vi "Rachel_Wheel_TestV2.vi"(10 "Spin or not to spin":bool, 11 "Oculus Data":T1={"head"={"orientation"={"roll"=1.6327005330047937, "pitch"=-89.08559793078238, "yaw"=-40.95061142092874}, "position"={"x"=1.207441, "y"=0.483058, "z"=-0.742013}}, "hands"={"left"={"position"={"x"=inf, "y"=inf, "z"=-inf}, "orientation"={"roll"=-51.475846117481964, "pitch"=106.93248840397386, "yaw"=69.74254276716579}}, "right"={"position"={"x"=inf, "y"=inf, "z"=-inf}, "orientation"={"roll"=49.02272731762935, "pitch"=105.46319543414037, "yaw"=-123.9602784132463}}}, "buttons"={"a"=FALSE, "b"=FALSE, "x"=FALSE, "y"=FALSE, "menu"=FALSE, "leftTrig"=1e-06, "rightTrig"=1e-06, "leftGrip"=1e-06, "rightGrip"=1e-06, "left_jstick"={"x"=-0.002561, "y"=0.007201, "button"=FALSE}, "right_jstick"={"x"=0.0, "y"=0.0, "button"=FALSE}}}) -> (3 "2D Picture":picture)   [LabVIEW 2017]
uses:
  <vilib>/myRIO/Instrument Drivers/Onboard IO/PWM/typedefs/PWM Reference.ctl
  <vilib>/myRIO/Common/Instrument Driver Framework/Utilities/typedefs/myRIO Generic Hardware Reference.ctl
  <vilib>/myRIO/Common/Instrument Driver Framework/Utilities/typedefs/Hardware Version Enum.ctl
  <vilib>/myRIO/Common/Instrument Driver Framework/Utilities/typedefs/myRIO v1.0 Reference.ctl
  <vilib>/myRIO/Common/Instrument Driver Framework/Utilities/typedefs/Generic FPGA Reference.ctl
  <vilib>/myRIO/Common/Instrument Driver Framework/myRIO v1.0/PWM/typedefs/PWM Channels Enum.ctl
  <vilib>/myRIO/Instrument Drivers/Onboard IO/PWM/typedefs/PWM Configuration.ctl
  <vilib>/userdefined/High Color/nirio_resource_hc.ctl
  <vilib>/myRIO/Common/Instrument Driver Framework/Utilities/vis/Is FPGA Ref Available.vi
  <vilib>/myRIO/Common/Instrument Driver Framework/myRIO v1.0/PWM/vis/myRIO v1.1 Open PWM.vi
  <vilib>/myRIO/Instrument Drivers/Onboard IO/PWM/vis/Set Duty Cycle and Frequency.vi
  <vilib>/myRIO/Common/Instrument Driver Framework/Utilities/vis/Validate Channels.vi
  <vilib>/myRIO/Common/Instrument Driver Framework/myRIO v1.0/PWM/vis/myRIO v1.0 Reserve PWM.vi
  <vilib>/myRIO/Common/Instrument Driver Framework/myRIO v1.0/PWM/vis/myRIO v1.0 Build MUX Configuration PWM.vi
  <vilib>/myRIO/Common/Instrument Driver Framework/myRIO v1.0/Resource Manager/vis/myRIO v1.0 Reserve Channel List.vi
  <vilib>/myRIO/Common/Instrument Driver Framework/myRIO v1.0/Resource Manager/vis/myRIO v1.0 Create Configuration List.vi
  <vilib>/myRIO/Common/Instrument Driver Framework/myRIO v1.0/Resource Manager/vis/myRIO v1.0 Reserve Channel.vi
  <vilib>/myRIO/Common/Instrument Driver Framework/myRIO v1.0/Resource Manager/vis/myRIO v1.0 Unreserve Channel.vi
  <vilib>/myRIO/Common/Instrument Driver Framework/myRIO v1.0/Resource Manager/vis/myRIO v1.0 Build Mutex Name.vi
  <vilib>/Utility/VariantDataType/GetNumericInfo.vi
  <vilib>/Utility/error.llb/Error Cluster From Error Code.vi
  <vilib>/myRIO/Common/Instrument Driver Framework/myRIO v1.0/myRIO v1.1 Open.vi
  <vilib>/myRIO/Common/Instrument Driver Framework/Utilities/vis/IO Manager.vi
  <vilib>/myRIO/Common/Instrument Driver Framework/Utilities/vis/Configuration Manager.vi
  <vilib>/myRIO/Common/Instrument Driver Framework/myRIO v1.0/Resource Manager/vis/myRIO v1.0 Configure IO.vi
  <vilib>/myRIO/Common/Instrument Driver Framework/myRIO v1.0/myRIO v1.0 Close.vi
  <vilib>/myRIO/Common/Instrument Driver Framework/myRIO v1.0/PWM/vis/myRIO v1.0 Write PWM.vi
  <vilib>/express/express arith-compare/Formula/XNode/ExpressFormulaBlockNode.xnode
  <vilib>/myRIO/Express VI/Onboard IO/PWM/PWM Express VI.xnode
  <vilib>/myRIO/Instrument Drivers/Onboard IO/PWM/vis/myRIO PWM Open.xnode
  <vilib>/myRIO/Instrument Drivers/Onboard IO/PWM/PWM.lvlib
panel:
  out "output cluster 2":cluster{dbl, dbl}={149.4878, 198.5598}
  in  "Arrow Size":dbl=15.0 format="%#_13g"
  in  "Rotation Radius":dbl=50.0 format="%#_13g"
  out "max value":dbl=0.007516748932651743
  out "SuMM":dbl(slide)=2.168404344971009e-18 scale=-3.0..3.0
  out "M3 Slider":dbl(slide)=-0.004955748932651739 scale=-1.0..1.0
  out "M2 Slider":dbl(slide)=0.007516748932651743 scale=-1.0..1.0
  out "M1 Slider":dbl(slide)=-0.002561000000000002 scale=-1.0..1.0
  out "r scaled":dbl=0.007642847767684503
  out "Duty 3":dbl=0.075
  out "Duty 2":dbl=0.075
  out "Duty 1":dbl=0.075
  out "buttons.rightGrip":dbl=1e-06
  out "buttons.leftGrip":dbl=1e-06
  out "RightJoyStick X":dbl(slide) scale=-1.0..1.0
  out "X":dbl=-0.002561
  out "theta temp":dbl=1.91249126492638
  out "r":dbl=0.007642847767684503
  out "M 3":dbl=-0.004955748932651739
  out "M 2":dbl=0.007516748932651743
  out "M 1":dbl=-0.002561000000000002
  out "Theta3":dbl=220.4223221640822
  out "Theta2":dbl=100.4223221640822
  out "Theta1":dbl=-19.577677835917797
  out "output cluster":cluster{dbl, dbl}={199.4878, 198.5598}
  out "Phi":dbl=109.5776778359178
  out "alpha3":dbl=330.0
  out "alpha2":dbl=210.0
  out "alpha1":dbl=90.0
  out "Y":dbl=0.007201
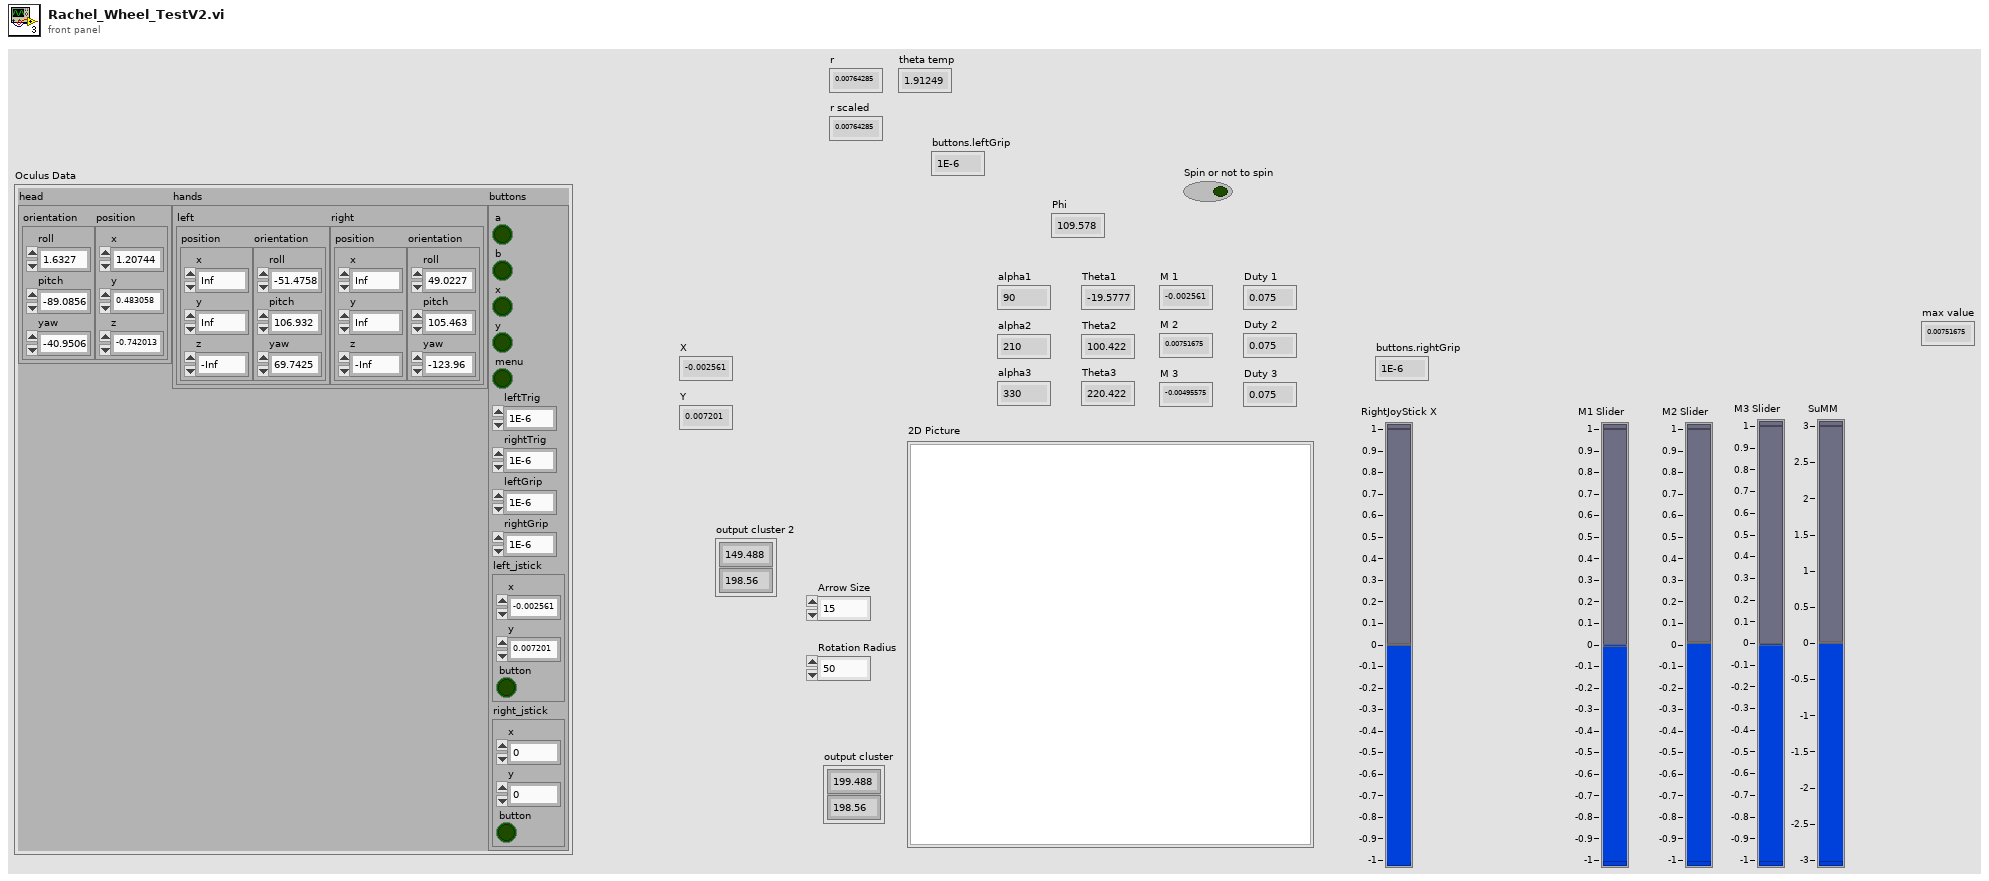
[diagram p1: front panel]
types:
  T1 = cluster{"head":cluster{"orientation":cluster{"roll":dbl, "pitch":dbl, "yaw":dbl}, "position":cluster{"x":dbl, "y":dbl, "z":dbl}}, "hands":cluster{"left":cluster{"position":cluster{"x":dbl, "y":dbl, "z":dbl}, "orientation":cluster{"roll":dbl, "pitch":dbl, "yaw":dbl}}, "right":cluster{"position":cluster{"x":dbl, "y":dbl, "z":dbl}, "orientation":cluster{"roll":dbl, "pitch":dbl, "yaw":dbl}}}, "buttons":cluster{"a":bool, "b":bool, "x":bool, "y":bool, "menu":bool, "leftTrig":dbl, "rightTrig":dbl, "leftGrip":dbl, "rightGrip":dbl, "left_jstick":cluster{"x":dbl, "y":dbl, "button":bool}, "right_jstick":cluster{"x":dbl, "y":dbl, "button":bool}}}
  T2 = cluster{"left":i16, "top":i16, "right":i16, "bottom":i16}
  T3 = cluster{"Width":u16, "Style":enum32{"Solid", "Dash", "Dot", "DashDot", "DashDotDot"}}
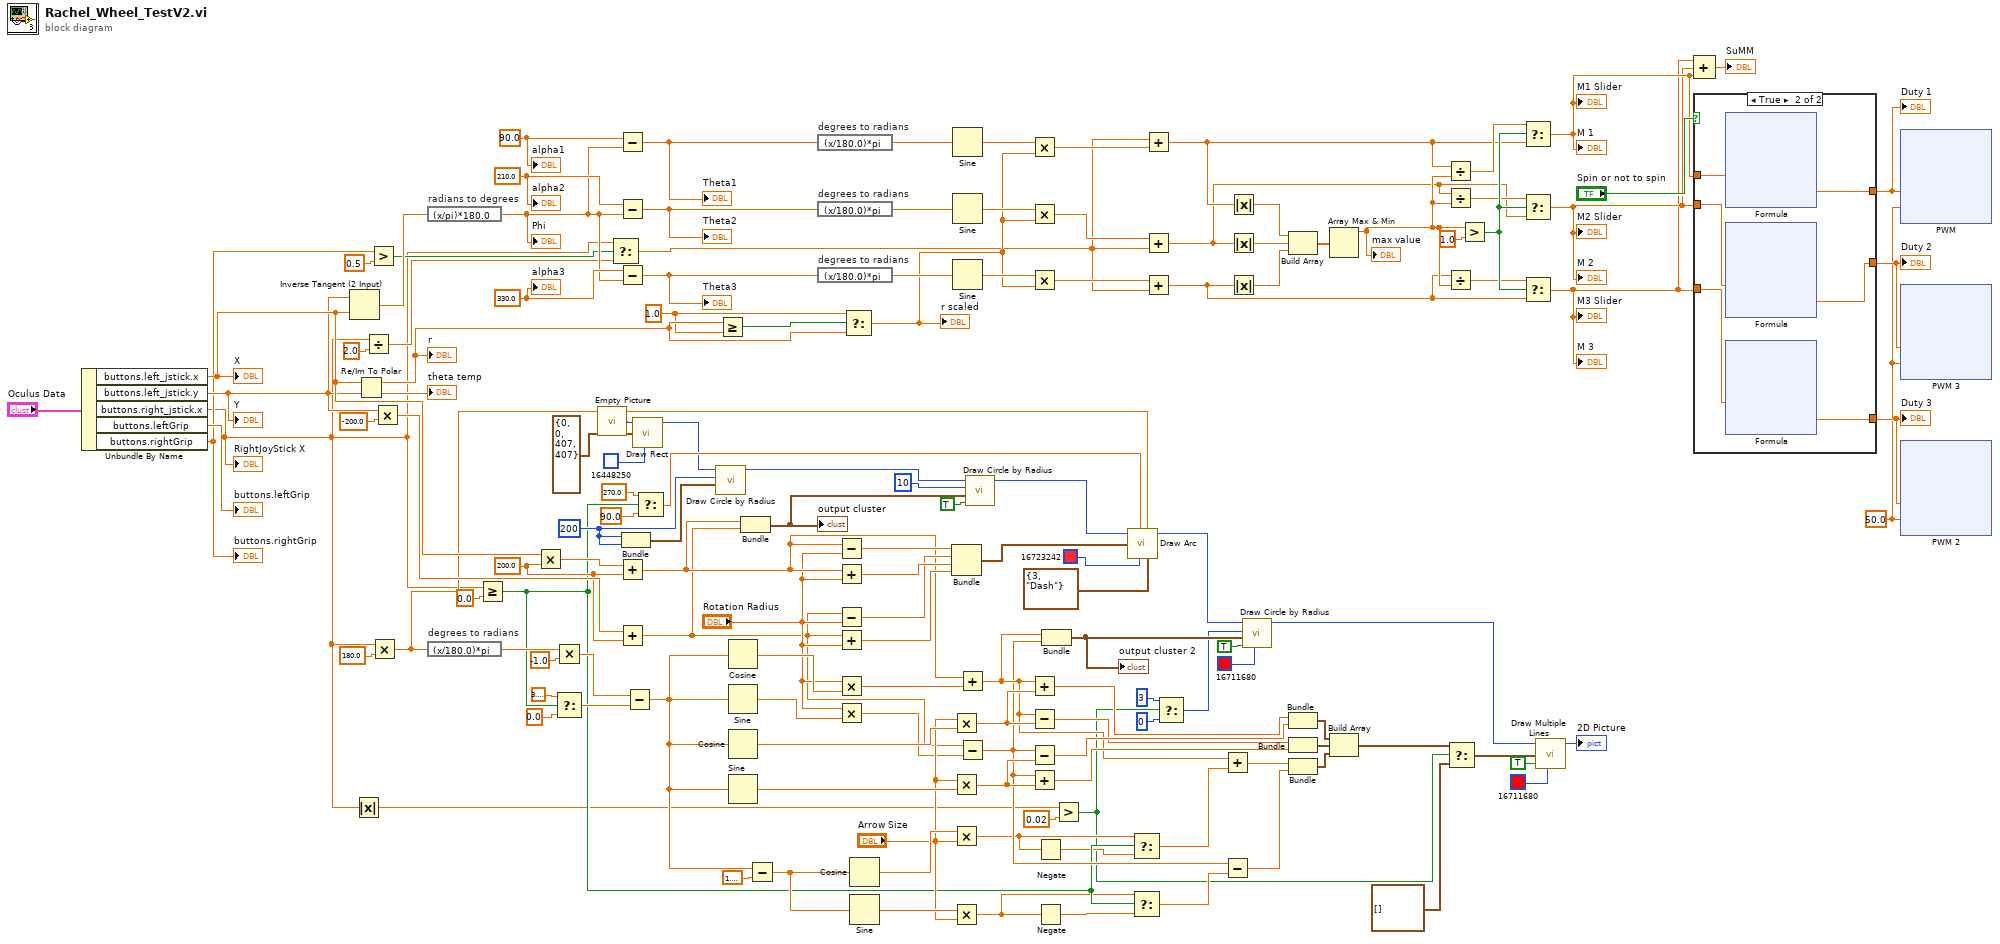
[diagram p0: block diagram]
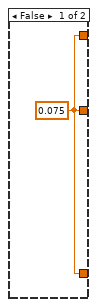
[diagram p2: hidden frame]
diagram:
  w104 = 50.0 ("y")
  w107 = 1.0 ("t")
  w135 = 200.0 ("y")
  w140 = i16 200 ("radius")
  w128 = 330.0 ("y")
  w129 = 210.0 ("y")
  w130 = 90.0 ("y")
  n1 = Unbundle By Name("Oculus Data") -> ("buttons.left_jstick.x"=w116:dbl, "buttons.left_jstick.y"=w115:dbl, "buttons.right_jstick.x"=w8:dbl, "buttons.leftGrip"=→"buttons.leftGrip":dbl, "buttons.rightGrip"=w102:dbl)
  "Y" <- w115
  "X" <- w116
  "RightJoyStick X" <- w8
  "buttons.rightGrip" <- w102
  n2 = Inverse Tangent (2 Input)(1:w116, 2:w115) -> (0:w141:dbl)
  n3 = Absolute Value(x=w8) -> (abs(x)=w10:dbl)
  n4 = Re/Im To Polar(2:w115, 3:w116) -> (0:→"theta temp":dbl, 1:w108:dbl)
  "r" <- w108
  n5 = Divide(x=w8, y=2.0) -> (x/y=w80:dbl)
  n6 = Greater?(x=w102, y=0.5) -> (0:w22:bool)
  n7 = Multiply(x=w8, y=180.0) -> (x*y=w40:dbl)
  n8 = Multiply(x=w115, y=-200.0) -> (x*y=w137:dbl)
  n9 = expression code="(x/pi)*180.0" "radians to degrees"(w141) -> (w127:dbl)
  "Phi" <- w127
  n10 = expression code="(x/180.0)*pi" "degrees to radians"(w40) -> (w35:dbl)
  n11 = Greater Or Equal?(x=w8, y=0.0) -> (x >= y?=w18:bool)
  n12 = Multiply(x=w116, y=w135) -> (x*y=w138:dbl)
  n13 = Multiply(x=w35, y=-1.0) -> (x*y=w33:dbl)
  n14 = Select(t=3.141592653589793, s=w18, f=0.0) -> (s? t:f=w21:dbl)
  n15 = call "Empty Picture"() -> ("empty picture"=w65:picture)
  n16 = Select(t=w8, s=w22, f=w80) -> (s? t:f=w97:dbl)
  n17 = Subtract(x=w130, y=w127) -> (x-y=w124:dbl)
  "Theta1" <- w124
  n18 = Subtract(x=w129, y=w127) -> (x-y=w126:dbl)
  "Theta2" <- w126
  n19 = Subtract(x=w128, y=w127) -> (x-y=w125:dbl)
  "Theta3" <- w125
  n20 = Add(x=w138, y=w135) -> (x+y=w41:dbl)
  n21 = Add(x=w137, y=w135) -> (x+y=w32:dbl)
  n22 = Bundle("radius"=w140, "radius"=w140) -> (w139:cluster{"radius":i16, "radius":i16})  [unwired: 1 in]
  n23 = Subtract(x=w33, y=w21) -> (x-y=w23:dbl)
  n24 = call <vilib>:"Draw Rect.vi"("picture"=w65, "rect"=T2 {"left"=0, "top"=0, "right"=407, "bottom"=407}, "color(black)"=u32 16448250) -> ("new picture"=w66:picture)  [unwired: 6 in]
  n25 = Select(t=270.0, s=w18, f=90.0) -> (s? t:f=w75:dbl)
  n26 = call <vilib>:"Draw Circle by Radius.vi"("pixel center"=w139, "radius"=w140, "picture"=w66) -> ("new picture"=w134:picture)  [unwired: 8 in]
  n27 = Greater Or Equal?(x=w108, y=w107) -> (x >= y?=w109:bool)
  n28 = Cosine(x=w23) -> (cos(x)=w39:dbl)
  n29 = Sine(x=w23) -> (sin(x)=w38:dbl)
  n30 = Cosine(x=w23) -> (cos(x)=w61:dbl)
  n31 = Sine(x=w23) -> (sin(x)=w55:dbl)
  n32 = Bundle(w41, w32) -> (w132:cluster{dbl, dbl})  [unwired: 1 in]
  "output cluster" <- w132
  n33 = Subtract(x=w23, y=1.5707963267948966) -> (x-y=w47:dbl)
  n34 = expression code="(x/180.0)*pi" "degrees to radians"(w124) -> (w122:dbl)
  n35 = expression code="(x/180.0)*pi" "degrees to radians"(w126) -> (w120:dbl)
  n36 = expression code="(x/180.0)*pi" "degrees to radians"(w125) -> (w118:dbl)
  n37 = Subtract(x=w41, y="Rotation Radius") -> (x-y=w71:dbl)
  n38 = Add(x=w41, y="Rotation Radius") -> (x+y=w70:dbl)
  n39 = Subtract(x=w32, y="Rotation Radius") -> (x-y=w69:dbl)
  n40 = Add(x=w32, y="Rotation Radius") -> (x+y=w68:dbl)
  n41 = Multiply(x="Rotation Radius", y=w39) -> (x*y=w36:dbl)
  n42 = Multiply(x="Rotation Radius", y=w38) -> (x*y=w31:dbl)
  n43 = Select(t=w107, s=w109, f=w108) -> (s? t:f=w110:dbl)
  "r scaled" <- w110
  n44 = Cosine(x=w47) -> (cos(x)=w45:dbl)
  n45 = Sine(x=w47) -> (sin(x)=w46:dbl)
  n46 = Bundle(w71, w69, w70, w68) -> (w67:cluster{dbl, dbl, dbl, dbl})  [unwired: 1 in]
  n47 = Multiply(x="Arrow Size", y=w61) -> (x*y=w53:dbl)
  n48 = Multiply(x="Arrow Size", y=w55) -> (x*y=w50:dbl)
  n49 = Multiply(x=w45, y="Arrow Size") -> (x*y=w12:dbl)
  n50 = Multiply(x=w46, y="Arrow Size") -> (x*y=w16:dbl)
  n51 = Sine(x=w122) -> (sin(x)=w123:dbl)
  n52 = Sine(x=w120) -> (sin(x)=w121:dbl)
  n53 = Sine(x=w118) -> (sin(x)=w119:dbl)
  n54 = Add(x=w41, y=w36) -> (x+y=w29:dbl)
  n55 = Subtract(x=w32, y=w31) -> (x-y=w28:dbl)
  n56 = call <vilib>:"Draw Circle by Radius.vi"("fill?(F)"=TRUE, "pixel center"=w132, "radius"=i16 10, "picture"=w134) -> ("new picture"=w79:picture)  [unwired: 7 in]
  n57 = Multiply(x=w123, y=w110) -> (x*y=w100:dbl)
  n58 = Multiply(x=w121, y=w110) -> (x*y=w99:dbl)
  n59 = Multiply(x=w119, y=w110) -> (x*y=w98:dbl)
  n60 = Add(x=w29, y=w53) -> (x+y=w56:dbl)
  n61 = Subtract(x=w29, y=w53) -> (x-y=w52:dbl)
  n62 = Subtract(x=w28, y=w50) -> (x-y=w54:dbl)
  n63 = Add(x=w28, y=w50) -> (x+y=w51:dbl)
  n64 = Negate(x=w12) -> (-x=w13:dbl)
  n65 = Negate(x=w16) -> (-x=w17:dbl)
  n66 = Bundle(w29, w28) -> (w27:cluster{dbl, dbl})  [unwired: 1 in]
  "output cluster 2" <- w27
  n67 = Greater?(x=w10, y=0.02 ("f")) -> (0:w7:bool)
  n68 = call <vilib>:"Draw Arc.vi"("picture"=w79, "start angle[degrees]"=w75, "rect"=w67, "color(black)"=u32 16723242, "arc size[degrees]"=w40, "pen"=T3 {"Width"=3, "Style"=enum."Dash"}) -> ("new picture"=w25:picture)  [unwired: 3 in]
  n69 = Select(t=w12, s=w18, f=w13) -> (s? t:f=w14:dbl)
  n70 = Select(t=w16, s=w18, f=w17) -> (s? t:f=w15:dbl)
  n71 = Add(x=w97, y=w100) -> (x+y=w86:dbl)
  n72 = Add(x=w99, y=w97) -> (x+y=w81:dbl)
  n73 = Add(x=w98, y=w97) -> (x+y=w82:dbl)
  n74 = Select(t=i16 3 ("radius"), s=w7, f=i16 0) -> (s? t:f=w3:i16)
  n75 = Add(x=w29, y=w14) -> (x+y=w42:dbl)
  n76 = Subtract(x=w28, y=w15) -> (x-y=w43:dbl)
  n77 = Absolute Value(x=w86) -> (abs(x)=w95:dbl)
  n78 = Absolute Value(x=w81) -> (abs(x)=w94:dbl)
  n79 = Absolute Value(x=w82) -> (abs(x)=w93:dbl)
  n80 = call <vilib>:"Draw Circle by Radius.vi"("color(black)"=u32 16711680, "fill?(F)"=TRUE, "pixel center"=w27, "radius"=w3, "picture"=w25) -> ("new picture"=w26:picture)  [unwired: 6 in]
  n81 = Build Array(w95, w94, w93) -> (w96:dbl[])
  n82 = Bundle(w56, w54) -> (w59:cluster{dbl, dbl})  [unwired: 1 in]
  n83 = Bundle(w52, w51) -> (w58:cluster{dbl, dbl})  [unwired: 1 in]
  n84 = Bundle(w42, w43) -> (w57:cluster{dbl, dbl})  [unwired: 1 in]
  n85 = Array Max & Min(array=w96) -> (max value=w83:dbl)  [unwired: 3 out]
  "max value" <- w83
  n86 = Build Array(w59, w58, w57) -> (w6:cluster{dbl, dbl}[])
  n87 = Divide(x=w86, y=w83) -> (x/y=w87:dbl)
  n88 = Divide(x=w81, y=w83) -> (x/y=w84:dbl)
  n89 = Divide(x=w82, y=w83) -> (x/y=w85:dbl)
  n90 = Select(t=w6, s=w7, f=cluster{"x":i16, "y":i16}[] [] ("line endpoints")) -> (s? t:f=w4:cluster{"x":dbl, "y":dbl}[])
  n91 = Greater?(x=w83, y=1.0) -> (0:w90:bool)
  n92 = Select(t=w87, s=w90, f=w86) -> (s? t:f=w91:dbl)
  "M 1" <- w91
  "M1 Slider" <- w91
  n93 = Select(t=w84, s=w90, f=w81) -> (s? t:f=w89:dbl)
  "M 2" <- w89
  "M2 Slider" <- w89
  n94 = Select(t=w85, s=w90, f=w82) -> (s? t:f=w88:dbl)
  "M 3" <- w88
  "M3 Slider" <- w88
  n95 = call <vilib>:"Draw Multiple Lines.vi"("picture"=w26, "line endpoints"=w4, "fill?(F)"=TRUE, "color(black)"=u32 16711680) -> ("new picture"=→"2D Picture":picture)  [unwired: 5 in]
  n96 = Compound Arithmetic op=ADD(w88, w89, w91) -> (→"SuMM":dbl)
  n97 = case shown="True" "Spin or not to spin" {
    tunnel: [w142 w148] -> w113
    tunnel: [w142 w147] -> w112
    tunnel: [w142 w146] -> w111
    tunnel: w88 -> [_ w145]
    tunnel: w89 -> [_ w144]
    tunnel: w91 -> [_ w143]
    frame False {
      w142 = 0.075
    }
    frame True {
      n98 = xnode "Formula"("X1"=w143) -> ("Result"=w148:dbl)  [unwired: 1 in, 1 out]
      n99 = xnode "Formula"("X1"=w144) -> ("Result"=w146:dbl)  [unwired: 1 in, 1 out]
      n100 = xnode "Formula"("X1"=w145) -> ("Result"=w147:dbl)  [unwired: 1 in, 1 out]
    }
  }
  "Duty 1" <- w113
  "Duty 2" <- w111
  "Duty 3" <- w112
  n101 = xnode "PWM"("Duty Cycle"=w113, "Frequency [Hz]"=w104) -> ()  [unwired: 1 in, 1 out]
  n102 = xnode "PWM 3"("Duty Cycle"=w111, "Frequency [Hz]"=w104) -> ()  [unwired: 1 in, 1 out]
  n103 = xnode "PWM 2"("Duty Cycle"=w112, "Frequency [Hz]"=w104) -> ()  [unwired: 1 in, 1 out]
  "alpha1" <- w130
  "alpha2" <- w129
  "alpha3" <- w128
